vi "Controle_Manip_Main_GUI_Backup0.vi"() -> ()   [LabVIEW 2019]
doc: "VI for micro-photoluminescence setup in GH013 to study the emission properties of single nanoemitters in the visible range."
uses:
  Desktop/Manip_uPL_visible_2020/SubVIs/ExistingSetupVIs/Setup_L065/Ligth Field/lightfield-automation-labview/LightField Automation.lvclass
  Desktop/Manip_uPL_visible_2020/SubVIs/ExistingSetupVIs/GH014/Labview/ESP 301/Newport ESP301/Newport ESP301.lvlib
panel:
  in  "Acq Time (ms)":dbl=500.0 caption="Acq Time" min=0.0 max=360000.0 step=50.0
  in  "Auto< ?":bool
  in  "Acq Mode":T1(ring) caption="Acq mode"
  in  "Shutter open":bool
  in  "Comment":string
  out "Log file":string caption="Status"
  in  "Experiment Name":string="B1802CF_QD0"
  in  "Experiment Graph Controls":T2(tab)
  in  "Acquire Continuous Spectrum":bool
  in  "Acquire Spectrum":bool
  out "CCD 2D Image Main":dbl[][](graph)
  in  "Save Spectrum N":bool
  in  "Save Spectrum":bool
  out "CCD 1D Spectrum Main":dbl[](graph)
  out "XY Intensity Map":dbl[][](graph)
  out "CCD 2D Image XY Map":dbl[][](graph)
  out "CCD 1D Spectrum XY Map":dbl[](graph)
  out "Polarisation 2D Image":dbl[][](graph)
  in  "Excitation Wavelength (nm)":dbl=400.0 caption="Exc WL (nm)" min=400.0 max=1100.0 step=1.0
  out "Photodiode Status":bool caption="Status"
  in  "Photodiode COM Port":refnum<visa-resource-name>="COM1" caption="COM Port"
  in  "ESP 301 COM Port":refnum<visa-resource-name>="COM4" caption="COM Port"
  in  "FSM Y Axis":tag
  in  "FSM X Axis":tag
  in  "Stop photodiode":bool
  in  "RotStage Exc Velocity":dbl=2.0 caption="Exc Velocity (°/s)"
  in  "RotStage Det Velocity":dbl=2.0 caption="Det Velocity (°/s)"
  in  "Camera Choice":u16
  out "LightField Automation out":refnum<class "LightField Automation.lvclass">
  in  "Slit Width (mm)":dbl
  out "Visible":bool
  out "Params CCD":string
  in  "Stop Everything & Quit?":bool
  in  "Excitation Source":enum16{"P", "CW"}(ring)=enum."CW" caption="Laser"
  in  "Temperature (K)":dbl=5.0 caption="T ="
  out "Excitation Power (uW)":dbl=0.2 caption="P    ="
  in  "Experimental parameters tab":T3(tab)
  in  "Spectrum Step Wavelength (nm)":dbl=490.12 caption="Step WL (nm)"
  in  "Spectrum End Wavelength (nm)":dbl=490.12 caption="End WL (nm)"
  in  "Spectrum Start Wavelength (nm)":dbl=490.12 caption="Start WL (nm)"
  in  "Accumulations":dbl=1.0 caption="Accum."
  in  "Background substract":enum16{"None", "Shutter"}(ring) caption="Bkg substract"
  in  "Exit mirror":enum16{"CCD", "APD"}(ring)
  in  "Center Wavelength (nm)":dbl=490.12 caption="Center WL (nm)"
  in  "Exposure Time (ms)":dbl=500.0 caption="Exp Time (ms)" min=0.0 max=360000.0 step=50.0
  in  "Grating":string(combo)
  in  "Scan Y Tot. Length":dbl caption="Y Length"
  in  "Scan X Tot. Length (V)":dbl caption="X Length (V)"
  in  "Scan Y Num. Pts":dbl caption="Y # Pts"
  in  "Scan X Num. Pts":dbl caption="X # Pts"
  in  "Scan Y Res. (V)":dbl caption="Res. Y (V)"
  in  "Scan X Res. (V)":dbl caption="Res. X (V)"
  in  "Scan Y Center (V)":dbl caption="Y Center (V)"
  in  "Scan X Center (V)":dbl caption="X Center (V)"
  in  "FSM Home":bool
  in  "FSM Right":bool
  in  "FSM Left":bool
  in  "FSM Down":bool
  in  "FSM Up":bool
  in  "FSM X Axis Pos":dbl
  in  "FSM Y Axis Pos":dbl
  in  "FSM Axis Step":dbl=0.1
  in  "Save XY Map":bool
  in  "Acquire XY Map":bool
  in  "Scanning Mode":T4(ring) caption="Mode"
  in  "Scan Fast Axis":enum16{"Y", "X"}(ring)=enum."X" caption="Fast Axis"
  in  "Acquire Polarisation":bool
  in  "RotStage Det Angle Target(°)":dbl=2.0 caption="Target (°)"
  in  "RotStage Exc Angle Target (°)":dbl=2.0 caption="Target (°)"
  in  "RotStage Det Angle Step (°)":dbl=2.0 caption="Step (°)"
  in  "RotStage Exc Angle Step (°) 2":dbl=2.0 caption="Step (°)"
  in  "RotStage Det Jog Forward":bool
  in  "RotStage Exc JogForward":bool
  in  "RotStage Det Jog Backward":bool
  in  "RotStage Det Home":bool caption="Home"
  in  "RotStage Exc Home":bool caption="Home"
  out "RotStage Det Angle (°)":dbl=2.0 caption="Readout (°)"
  out "RotStage Exc Angle (°)":dbl=2.0 caption="Readout (°)"
  in  "RotStage Exc Jog Backward":bool
  in  "Polar Start Angle (°)":dbl caption="Start angle (°)" min=0.0 max=360.0 step=10.0
  in  "Polar End Angle (°)":dbl=360.0 caption="End Angle (°)" min=0.0 max=360.0 step=10.0
  in  "Polar Step Angle (°)":dbl=10.0 caption="Step Angle (°)" min=1.0 max=360.0
  in  "Polar mode":enum16{"Excitation", "Detection"}(ring)=enum."Detection" caption="Rotate polarisation"
  in  "Save Polarisation":bool
  # "ms"
  # "Shutter"
  # "K"
  # "laser"
  # "uW"
  # "exc"
  # "Thorlabs PM16-120"
  # "Newport ESP 301 Controller"
  # "Controls"
  # "Scans"
  # "add functionnality spectrum with APD 1 or APD 2\nwith option AcqMode"
  # "Possibly add a slit size option to determine the resolution"
  # "Controls"
  # "Scans"
  # "Controls"
  # "Scans"
  # "Excitation"
  # "Jog"
  # "Go to"
  # "Detection"
  # "Controls"
  # "Scans"
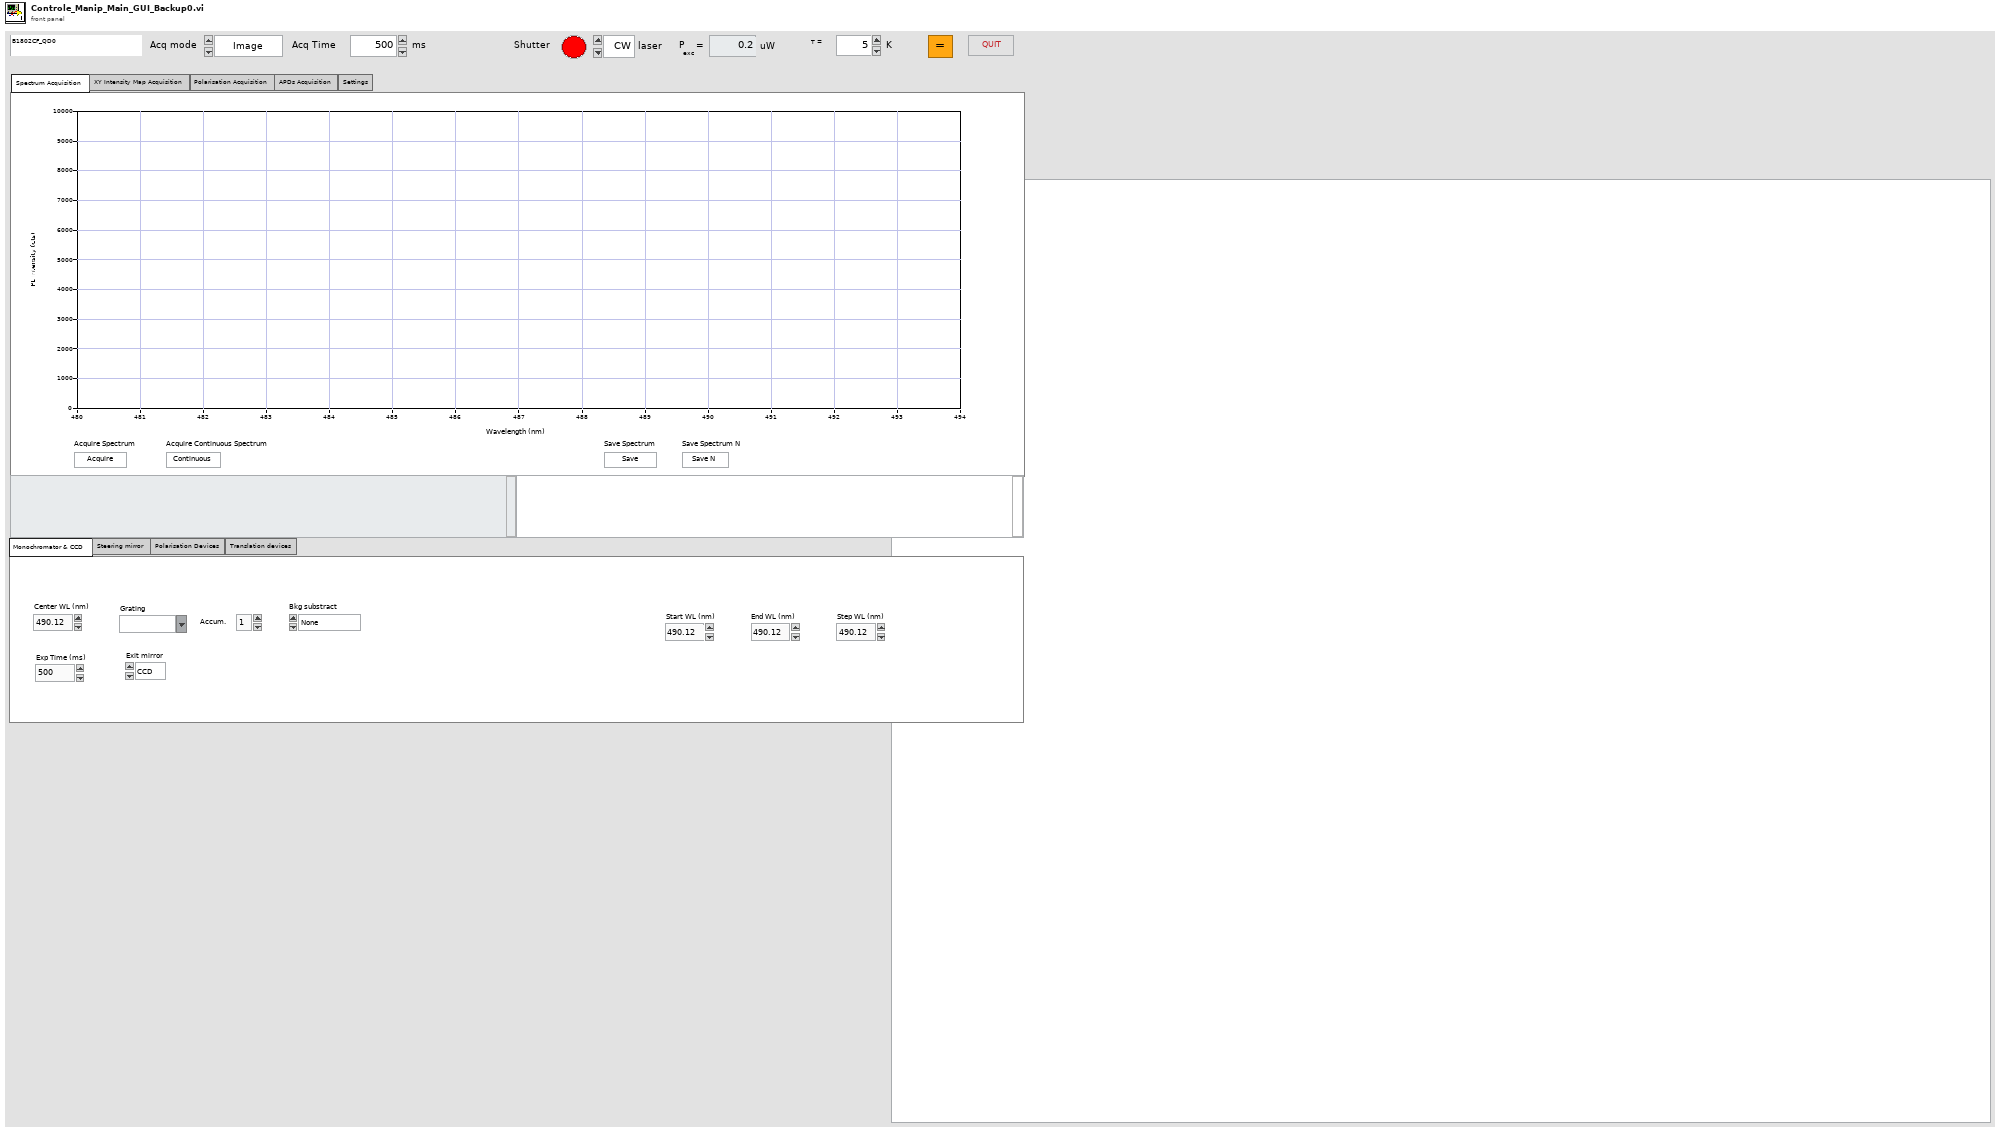
[diagram p1: front panel]
types:
  T1 = enum16{"Image", "Spectrum", "APD 1", "APD 2", "APD 1+2"}
  T2 = enum32{"Spectrum Acquisition", "XY Intensity Map Acquisition", "Polarisation Acquisition", "APDs Acquisition", "Settings"}
  T3 = enum32{"Monochromator & CCD", "Steering mirror", "Polarisation Devices", "Translation devices"}
  T4 = enum16{"Default", "Snail", "Random", "Snake", "Line"}
  T5 = enum16{"XY Intensity Map", "Polarisation", "Spectrum"}
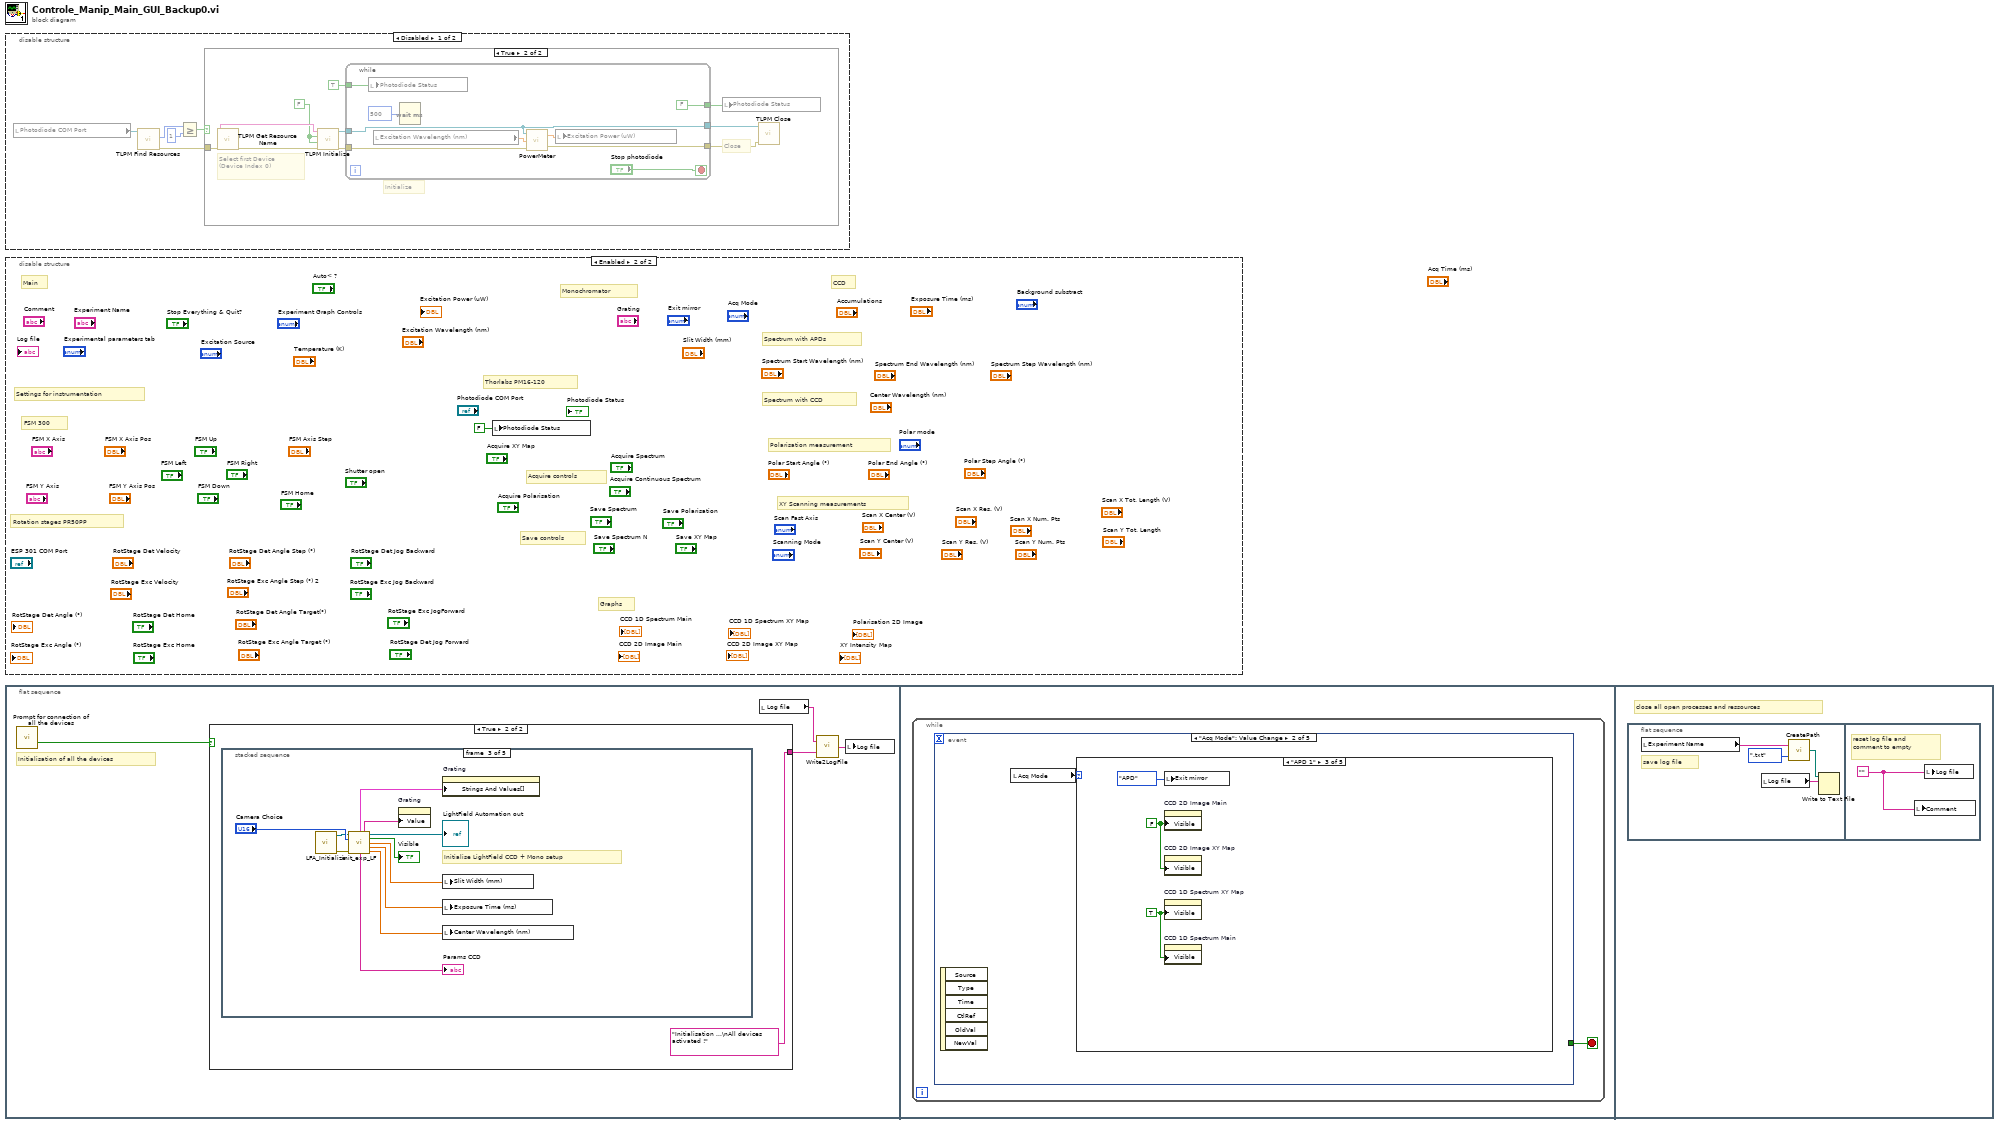
[diagram p0: block diagram]
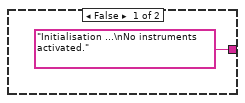
[diagram p5: hidden frame]
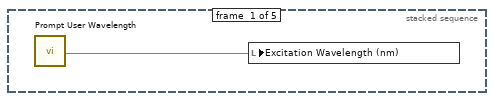
[diagram p6: hidden frame]
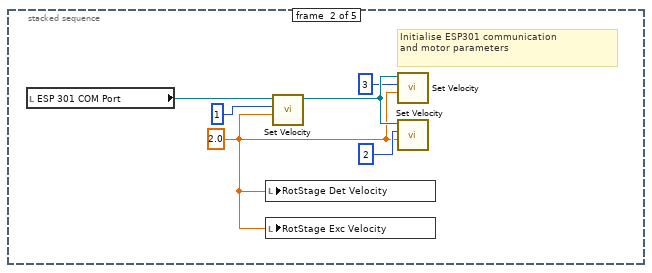
[diagram p7: hidden frame]
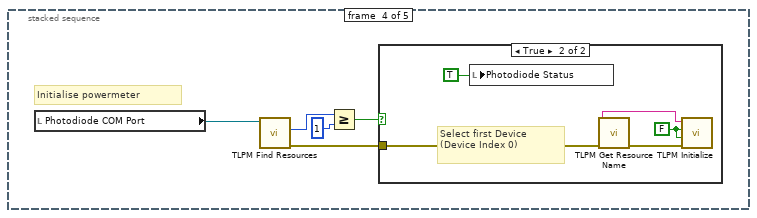
[diagram p8: hidden frame]
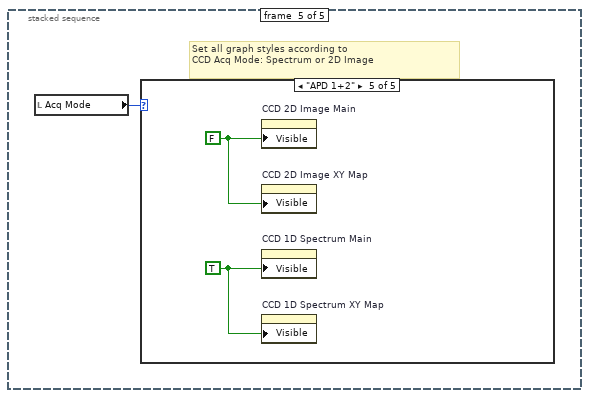
[diagram p10: hidden frame]
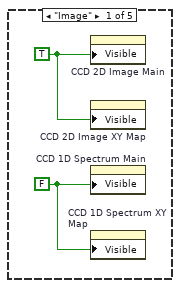
[diagram p11: hidden frame]
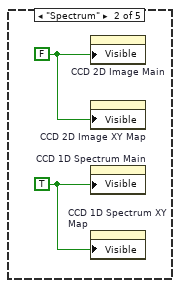
[diagram p12: hidden frame]
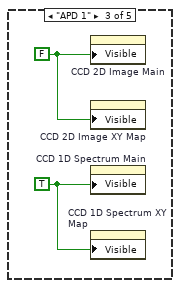
[diagram p13: hidden frame]
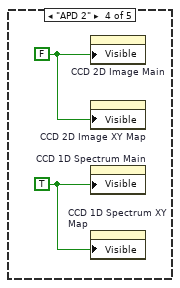
[diagram p14: hidden frame]
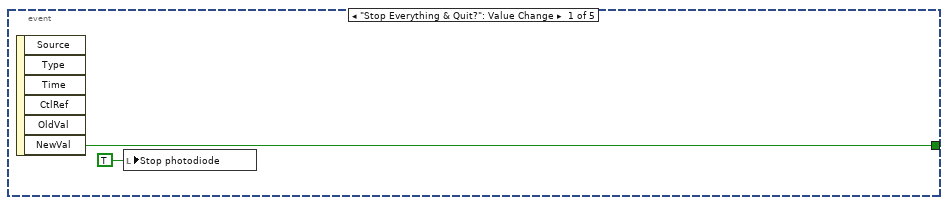
[diagram p15: hidden frame]
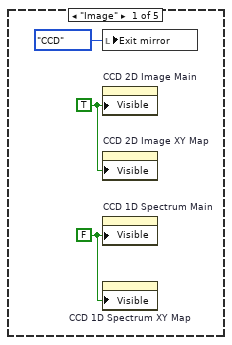
[diagram p16: hidden frame]
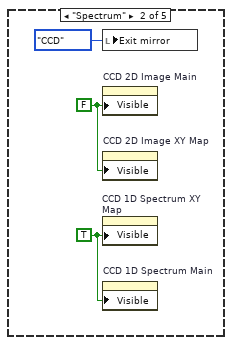
[diagram p17: hidden frame]
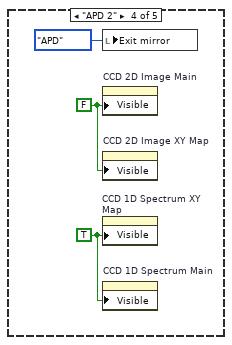
[diagram p18: hidden frame]
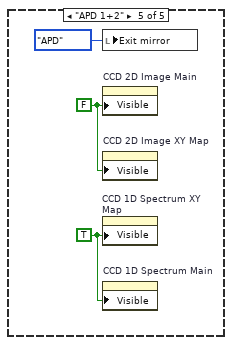
[diagram p19: hidden frame]
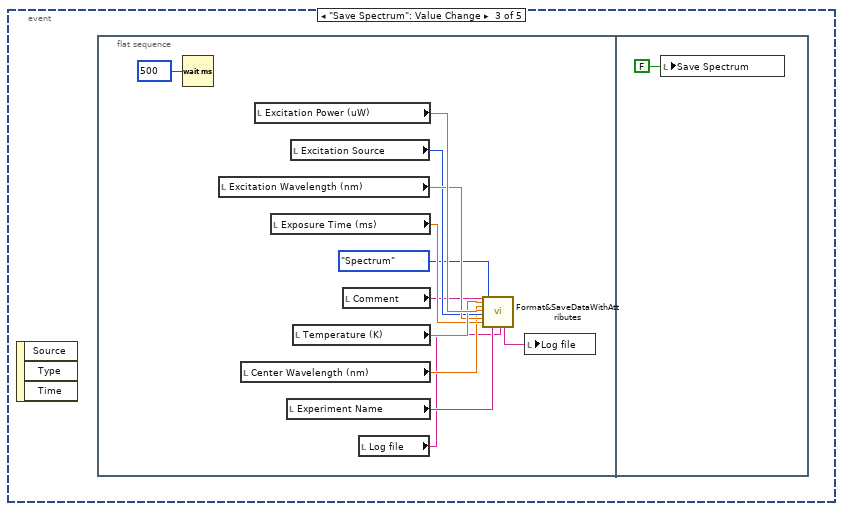
[diagram p20: hidden frame]
diagram:
  n1 = disable-structure shown="Disabled" {
    frame Disabled {
      n2 = local read "Photodiode COM Port"() -> (w5:refnum<visa-resource-name>)
      n3 = call <instrlib>:"TLPM Find Resources.vi"("instrument handle"=w5) -> ("error out"=w1:errorcluster, "Resource Count"=w4:u32)  [unwired: 8 in, 1 out]
      n4 = Greater Or Equal?(x=w4, y=1) -> (x >= y?=w2:bool)
      n5 = case shown="True" w2 {
        tunnel: w1 -> [_ w15]
        frame False {
        }
        frame True {
          w13 = FALSE
          # "Close"
          # "Initialize"
          # "Select first Device\n(Device Index 0)"
          n6 = call <instrlib>:"TLPM Get Resource Name.vi"("error in (no error)"=w15) -> ("error out"=w10:errorcluster, "Resource Name"=w14:string)  [unwired: 8 in, 1 out]
          n7 = call <instrlib>:"TLPM Initialize.vi"("error in (no error)"=w10, "Reset Device (Reset Device)"=w13, "ID Query (Do Query)"=w13, "resource name"=w14) -> ("error out"=w12:errorcluster, "instrument handle out"=w9:refnum<visa-resource-name>)  [unwired: 6 in]
          n8 = while {
            tunnel: w12 -> [w23]
            tunnel: TRUE -> [w24]
            tunnel: w9 -> [w20]
            tunnel: [w20] -> w8
            tunnel: [w19] -> w7
            tunnel: [FALSE] -> w6
            stop <- "Stop photodiode" stop-if-true
            n9 = local write "Photodiode Status"(w24) -> ()
            n10 = local read "Excitation Wavelength (nm)"() -> (w22:dbl)
            n11 = Wait (ms)(milliseconds to wait=u32 500) -> ()  [unwired: 1 out]
            n12 = call "PowerMeter.vi"("Error In"=w23, "Set Wavelength (nm)"=w22, "VISA resource name"=w20) -> ("Error Out"=w19:errorcluster, "Power Value"=w21:dbl)  [unwired: 1 in]
            n13 = local write "Excitation Power (uW)"(w21) -> ()
          }
          n14 = local write "Photodiode Status"(w6) -> ()
          n15 = call <instrlib>:"TLPM Close.vi"("error in (no error)"=w7, "instrument handle"=w8) -> ()  [unwired: 9 in, 1 out]
        }
      }
    }
    frame Enabled {
    }
  }
  n16 = disable-structure shown="Enabled" {
    frame Disabled {
    }
    frame Enabled {
      # "XY Scanning measurements"
      # "Polarisation measurement"
      # "Graphs"
      # "Spectrum with CCD"
      # "Spectrum with APDs"
      # "Acquire controls"
      # "Save controls"
      # "CCD"
      # "Monochromator"
      # "Rotation stages PR50PP"
      # "Main"
      # "Thorlabs PM16-120"
      # "FSM 300"
      # "Settings for instrumentation"
      n17 = local write "Photodiode Status"(FALSE) -> ()
    }
  }
  n18 = flat-sequence {
    frame #0 {
      # "Initialisation of all the devices"
      n19 = call "Prompt for connection of all the devices"() -> ("OK"=w29:bool)  [unwired: 18 in, 1 out]
      n20 = case shown="True" w29 {
        tunnel: ["Initialisation ...\nNo instruments activated." "Initialisation ...\nAll devices activated !"] -> w27
        frame False {
        }
        frame True {
          n21 = stacked-sequence {
            frame #0 {
              n22 = call "Prompt User Wavelength"() -> ("Wavelength"=w32:dbl)  [unwired: 17 in, 2 out]
              n23 = local write "Excitation Wavelength (nm)"(w32) -> ()
            }
            frame #1 {
              w33 = 2.0 ("Velocity (units/s)")
              # "Initialise ESP301 communication\nand motor parameters"
              n24 = local read "ESP 301 COM Port"() -> (w34:refnum<visa-resource-name>)
              n25 = local write "RotStage Det Velocity"(w33) -> ()
              n26 = local write "RotStage Exc Velocity"(w33) -> ()
              n27 = call "Set Velocity.vi"("Velocity (units/s)"=w33, "Axis (1)"=1, "VISA resource name"=w34) -> ("VISA resource name out"=w37:refnum<visa-resource-name>)  [unwired: 3 in, 1 out]
              n28 = call "Set Velocity.vi"("Velocity (units/s)"=w33, "Axis (1)"=3, "VISA resource name"=w37) -> ()  [unwired: 3 in, 2 out]
              n29 = call "Set Velocity.vi"("Velocity (units/s)"=w33, "Axis (1)"=2, "VISA resource name"=w37) -> ()  [unwired: 3 in, 2 out]
            }
            frame #2 {
              # "Initialise LightField CCD + Mono setup"
              n30 = call "LFA_Initialize.vi"() -> ("error out"=w49:errorcluster, "LightField Automation out"=w47:refnum<class "LightField Automation.lvclass">)  [unwired: 10 in]
              n31 = call "init_exp_LF.vi"("LightField Automation in"=w47, "Camera Choice"="Camera Choice", "error in (no error)"=w49) -> ("Array"=w39:cluster{"format string":string, string}[], "format string"=w40:string, "LightField Automation out"=→"LightField Automation out":refnum<class "LightField Automation.lvclass">, "Visible"=→"Visible":bool, "Slit Width"=w42:dbl, "Exposure Time (s)"=w43:dbl, "Params CCD"=→"Params CCD":string, "Center Wavelenght"=w44:dbl)  [unwired: 4 in, 1 out]
              n32 = property on="Grating" class="CmbBox"("Value"=w40) -> ()  [unwired: 2 in, 2 out]
              n33 = property on="Grating" class="CmbBox"("Strings And Values[]"=w39) -> ()  [unwired: 2 in, 2 out]
              n34 = local write "Slit Width (mm)"(w42) -> ()
              n35 = local write "Exposure Time (ms)"(w43) -> ()
              n36 = local write "Center Wavelength (nm)"(w44) -> ()
            }
            frame #3 {
              # "Initialise powermeter"
              n37 = local read "Photodiode COM Port"() -> (w52:refnum<visa-resource-name>)
              n38 = call <instrlib>:"TLPM Find Resources.vi"("instrument handle"=w52) -> ("error out"=w50:errorcluster, "Resource Count"=w53:u32)  [unwired: 8 in, 1 out]
              n39 = Greater Or Equal?(x=w53, y=1) -> (x >= y?=w51:bool)
              n40 = case shown="True" w51 {
                tunnel: w50 -> [_ w59]
                frame False {
                }
                frame True {
                  w58 = FALSE ("Reset Device (Reset Device)")
                  # "Select first Device\n(Device Index 0)"
                  n41 = local write "Photodiode Status"(TRUE) -> ()
                  n42 = call <instrlib>:"TLPM Get Resource Name.vi"("error in (no error)"=w59) -> ("error out"=w56:errorcluster, "Resource Name"=w57:string)  [unwired: 8 in, 1 out]
                  n43 = call <instrlib>:"TLPM Initialize.vi"("error in (no error)"=w56, "Reset Device (Reset Device)"=w58, "ID Query (Do Query)"=w58, "resource name"=w57) -> ()  [unwired: 6 in, 2 out]
                }
              }
            }
            frame #4 {
              # "Set all graph styles according to \nCCD Acq Mode: Spectrum or 2D Image"
              n44 = local read "Acq Mode"() -> (w60:T1)
              n45 = case shown="\"APD 1+2\"" w60 {
                frame "Image" {
                  w62 = TRUE
                  w61 = FALSE
                  n46 = property on="CCD 2D Image Main" class="IntGraph (strict)"("Visible"=w62) -> ()  [unwired: 2 in, 2 out]
                  n47 = property on="CCD 2D Image XY Map" class="IntGraph (strict)"("Visible"=w62) -> ()  [unwired: 2 in, 2 out]
                  n48 = property on="CCD 1D Spectrum Main" class="WFGraph (strict)"("Visible"=w61) -> ()  [unwired: 2 in, 2 out]
                  n49 = property on="CCD 1D Spectrum XY Map" class="WFGraph (strict)"("Visible"=w61) -> ()  [unwired: 2 in, 2 out]
                }
                frame "Spectrum" {
                  w63 = FALSE
                  w64 = TRUE
                  n50 = property on="CCD 2D Image Main" class="IntGraph (strict)"("Visible"=w63) -> ()  [unwired: 2 in, 2 out]
                  n51 = property on="CCD 2D Image XY Map" class="IntGraph (strict)"("Visible"=w63) -> ()  [unwired: 2 in, 2 out]
                  n52 = property on="CCD 1D Spectrum Main" class="WFGraph (strict)"("Visible"=w64) -> ()  [unwired: 2 in, 2 out]
                  n53 = property on="CCD 1D Spectrum XY Map" class="WFGraph (strict)"("Visible"=w64) -> ()  [unwired: 2 in, 2 out]
                }
                frame "APD 1" {
                  w65 = FALSE
                  w66 = TRUE
                  n54 = property on="CCD 2D Image Main" class="IntGraph (strict)"("Visible"=w65) -> ()  [unwired: 2 in, 2 out]
                  n55 = property on="CCD 2D Image XY Map" class="IntGraph (strict)"("Visible"=w65) -> ()  [unwired: 2 in, 2 out]
                  n56 = property on="CCD 1D Spectrum Main" class="WFGraph (strict)"("Visible"=w66) -> ()  [unwired: 2 in, 2 out]
                  n57 = property on="CCD 1D Spectrum XY Map" class="WFGraph (strict)"("Visible"=w66) -> ()  [unwired: 2 in, 2 out]
                }
                frame "APD 2" {
                  w67 = FALSE
                  w68 = TRUE
                  n58 = property on="CCD 2D Image Main" class="IntGraph (strict)"("Visible"=w67) -> ()  [unwired: 2 in, 2 out]
                  n59 = property on="CCD 2D Image XY Map" class="IntGraph (strict)"("Visible"=w67) -> ()  [unwired: 2 in, 2 out]
                  n60 = property on="CCD 1D Spectrum Main" class="WFGraph (strict)"("Visible"=w68) -> ()  [unwired: 2 in, 2 out]
                  n61 = property on="CCD 1D Spectrum XY Map" class="WFGraph (strict)"("Visible"=w68) -> ()  [unwired: 2 in, 2 out]
                }
                frame "APD 1+2" {
                  w69 = FALSE
                  w70 = TRUE
                  n62 = property on="CCD 2D Image Main" class="IntGraph (strict)"("Visible"=w69) -> ()  [unwired: 2 in, 2 out]
                  n63 = property on="CCD 2D Image XY Map" class="IntGraph (strict)"("Visible"=w69) -> ()  [unwired: 2 in, 2 out]
                  n64 = property on="CCD 1D Spectrum Main" class="WFGraph (strict)"("Visible"=w70) -> ()  [unwired: 2 in, 2 out]
                  n65 = property on="CCD 1D Spectrum XY Map" class="WFGraph (strict)"("Visible"=w70) -> ()  [unwired: 2 in, 2 out]
                }
              }
            }
          }
        }
      }
      n66 = local read "Log file"() -> (w28:string)
      n67 = call "Write2LogFile.vi"("Add to log file"=w27, "Log file before"=w28) -> ("Log file after"=w26:string)
      n68 = local write "Log file"(w26) -> ()
    }
    frame #1 {
      n69 = while {
        stop <- w71 stop-if-true
        n70 = event shown="[1] \"Acq Mode\": Value Change" {
          selector: _ -> [_ _ _ _ _]
          dyn-events: _ -> [_ _ _ _ _]
          timeout: _ -> [_ _ _ _ _]
          tunnel: [w73 _ _ _ _] -> w71
          event "Stop Everything & Quit?": Value Change {
            n71 = event-data() -> ("NewVal"=w73:bool)  [unwired: 1 in, 5 out]
            n72 = local write "Stop photodiode"(TRUE) -> ()
          }
          event "Acq Mode": Value Change {
            n73 = event-data() -> ()  [unwired: 1 in, 6 out]
            n74 = local read "Acq Mode"() -> (w74:T1)
            n75 = case shown="\"APD 1\"" w74 {
              frame "Image" {
                w76 = TRUE
                w77 = FALSE
                n76 = local write "Exit mirror"(enum16{"CCD", "APD"}."CCD" ("Exit mirror")) -> ()
                n77 = property on="CCD 2D Image Main" class="IntGraph (strict)"("Visible"=w76) -> ()  [unwired: 2 in, 2 out]
                n78 = property on="CCD 2D Image XY Map" class="IntGraph (strict)"("Visible"=w76) -> ()  [unwired: 2 in, 2 out]
                n79 = property on="CCD 1D Spectrum Main" class="WFGraph (strict)"("Visible"=w77) -> ()  [unwired: 2 in, 2 out]
                n80 = property on="CCD 1D Spectrum XY Map" class="WFGraph (strict)"("Visible"=w77) -> ()  [unwired: 2 in, 2 out]
              }
              frame "Spectrum" {
                w80 = FALSE
                w79 = TRUE
                n81 = local write "Exit mirror"(enum16{"CCD", "APD"}."CCD" ("Exit mirror")) -> ()
                n82 = property on="CCD 2D Image Main" class="IntGraph (strict)"("Visible"=w80) -> ()  [unwired: 2 in, 2 out]
                n83 = property on="CCD 2D Image XY Map" class="IntGraph (strict)"("Visible"=w80) -> ()  [unwired: 2 in, 2 out]
                n84 = property on="CCD 1D Spectrum XY Map" class="WFGraph (strict)"("Visible"=w79) -> ()  [unwired: 2 in, 2 out]
                n85 = property on="CCD 1D Spectrum Main" class="WFGraph (strict)"("Visible"=w79) -> ()  [unwired: 2 in, 2 out]
              }
              frame "APD 1" {
                w83 = FALSE
                w82 = TRUE
                n86 = local write "Exit mirror"(enum16{"CCD", "APD"}."APD" ("Exit mirror")) -> ()
                n87 = property on="CCD 2D Image Main" class="IntGraph (strict)"("Visible"=w83) -> ()  [unwired: 2 in, 2 out]
                n88 = property on="CCD 2D Image XY Map" class="IntGraph (strict)"("Visible"=w83) -> ()  [unwired: 2 in, 2 out]
                n89 = property on="CCD 1D Spectrum XY Map" class="WFGraph (strict)"("Visible"=w82) -> ()  [unwired: 2 in, 2 out]
                n90 = property on="CCD 1D Spectrum Main" class="WFGraph (strict)"("Visible"=w82) -> ()  [unwired: 2 in, 2 out]
              }
              frame "APD 2" {
                w86 = FALSE
                w85 = TRUE
                n91 = local write "Exit mirror"(enum16{"CCD", "APD"}."APD" ("Exit mirror")) -> ()
                n92 = property on="CCD 2D Image Main" class="IntGraph (strict)"("Visible"=w86) -> ()  [unwired: 2 in, 2 out]
                n93 = property on="CCD 2D Image XY Map" class="IntGraph (strict)"("Visible"=w86) -> ()  [unwired: 2 in, 2 out]
                n94 = property on="CCD 1D Spectrum XY Map" class="WFGraph (strict)"("Visible"=w85) -> ()  [unwired: 2 in, 2 out]
                n95 = property on="CCD 1D Spectrum Main" class="WFGraph (strict)"("Visible"=w85) -> ()  [unwired: 2 in, 2 out]
              }
              frame "APD 1+2" {
                w89 = FALSE
                w88 = TRUE
                n96 = local write "Exit mirror"(enum16{"CCD", "APD"}."APD" ("Exit mirror")) -> ()
                n97 = property on="CCD 2D Image Main" class="IntGraph (strict)"("Visible"=w89) -> ()  [unwired: 2 in, 2 out]
                n98 = property on="CCD 2D Image XY Map" class="IntGraph (strict)"("Visible"=w89) -> ()  [unwired: 2 in, 2 out]
                n99 = property on="CCD 1D Spectrum XY Map" class="WFGraph (strict)"("Visible"=w88) -> ()  [unwired: 2 in, 2 out]
                n100 = property on="CCD 1D Spectrum Main" class="WFGraph (strict)"("Visible"=w88) -> ()  [unwired: 2 in, 2 out]
              }
            }
          }
          event "Save Spectrum": Value Change {
            n101 = event-data() -> ()  [unwired: 1 in, 3 out]
            n102 = flat-sequence {
              frame #0 {
                n103 = Wait (ms)(milliseconds to wait=u32 500) -> ()  [unwired: 1 out]
                n104 = local read "Excitation Wavelength (nm)"() -> (w99:dbl)
                n105 = local read "Center Wavelength (nm)"() -> (w95:dbl)
                n106 = local read "Excitation Power (uW)"() -> (w101:dbl)
                n107 = local read "Exposure Time (ms)"() -> (w97:dbl)
                n108 = local read "Experiment Name"() -> (w94:string)
                n109 = local read "Excitation Source"() -> (w98:enum16{"P", "CW"})
                n110 = local read "Temperature (K)"() -> (w100:dbl)
                n111 = local read "Comment"() -> (w93:string)
                n112 = local read "Log file"() -> (w91:string)
                n113 = call "Format&SaveDataWithAttributes.vi"("Comment"=w93, "Exp_Temperature_K"=w100, "Det_Mono1_CenterWL_nm"=w95, "Exc_ExcitationPower_uW"=w101, "Exc_ExcitationSource"=w98, "Exc_ExcitationWavelength_nm"=w99, "Det_AcqTime_ms"=w97, "Measurement type"=T5."Spectrum", "FileName"=w94, "Log File In"=w91) -> ("Log File Out"=w90:string)  [unwired: 16 in, 1 out]
                n114 = local write "Log file"(w90) -> ()
              }
              frame #1 {
                n115 = local write "Save Spectrum"(FALSE) -> ()
              }
            }
          }
          event "Auto< ?": Value Change {
            n116 = event-data() -> ("NewVal"=w103:bool)  [unwired: 1 in, 5 out]
            n117 = case shown="True" w103 {
              frame False {
                w104 = TRUE ("Visible")
                n118 = property on="Save Spectrum N" class="Bool"("Visible"=w104) -> ()  [unwired: 2 in, 2 out]
                n119 = property on="Save XY Map" class="Bool"("Visible"=w104) -> ()  [unwired: 2 in, 2 out]
                n120 = property on="Save Spectrum" class="Bool (strict)"("Visible"=w104) -> ()  [unwired: 2 in, 2 out]
                n121 = property on="Save Polarisation" class="Bool (strict)"("Visible"=w104) -> ()  [unwired: 2 in, 2 out]
              }
              frame True {
                w105 = FALSE ("Visible")
                n122 = property on="Save Spectrum N" class="Bool"("Visible"=w105) -> ()  [unwired: 2 in, 2 out]
                n123 = property on="Save XY Map" class="Bool"("Visible"=w105) -> ()  [unwired: 2 in, 2 out]
                n124 = property on="Save Spectrum" class="Bool (strict)"("Visible"=w105) -> ()  [unwired: 2 in, 2 out]
                n125 = property on="Save Polarisation" class="Bool (strict)"("Visible"=w105) -> ()  [unwired: 2 in, 2 out]
              }
            }
          }
          event "Save Polarisation": Value Change {
            n126 = event-data() -> ()  [unwired: 1 in, 6 out]
            n127 = flat-sequence {
              frame #0 {
                n128 = Wait (ms)(milliseconds to wait=u32 500) -> ()  [unwired: 1 out]
                n129 = local read "Excitation Wavelength (nm)"() -> (w115:dbl)
                n130 = local read "Center Wavelength (nm)"() -> (w112:dbl)
                n131 = local read "Excitation Power (uW)"() -> (w117:dbl)
                n132 = local read "Exposure Time (ms)"() -> (w113:dbl)
                n133 = local read "Experiment Name"() -> (w109:string)
                n134 = local read "Excitation Source"() -> (w114:enum16{"P", "CW"})
                n135 = local read "Temperature (K)"() -> (w116:dbl)
                n136 = local read "Comment"() -> (w110:string)
                n137 = local read "Log file"() -> (w106:string)
                n138 = call "Format&SaveDataWithAttributes.vi"("Comment"=w110, "Exp_Temperature_K"=w116, "Det_Mono1_CenterWL_nm"=w112, "Exc_ExcitationPower_uW"=w117, "Exc_ExcitationSource"=w114, "Exc_ExcitationWavelength_nm"=w115, "Det_AcqTime_ms"=w113, "Measurement type"=T5."Polarisation", "FileName"=w109, "Log File In"=w106) -> ("Log File Out"=w107:string)  [unwired: 16 in, 1 out]
                n139 = local write "Log file"(w107) -> ()
              }
              frame #1 {
                n140 = local write "Save Polarisation"(FALSE) -> ()
              }
            }
          }
        }
      }
    }
    frame #2 {
      # "close all open processes and ressources"
      n141 = flat-sequence {
        frame #0 {
          # "save log file"
          n142 = local read "Experiment Name"() -> (w121:string)
          n143 = local read "Log file"() -> (w122:string)
          n144 = call "CreatePath.vi"("filetype"=enum16{".h5", ".txt"}.".txt", "FileName"=w121) -> ("File path"=w119:path)
          n145 = Write to Text File(file (use dialog)=w119, text=w122) -> ()  [unwired: 2 in, 3 out]
        }
        frame #1 {
          w123 = ""
          # "reset log file and \ncomment to empty"
          n146 = local write "Comment"(w123) -> ()
          n147 = local write "Log file"(w123) -> ()
        }
      }
    }
  }
